vi "ROI grp-Recover Groups array setup.vi"(8 "error in (no error)":errorcluster) -> (0 "error out":errorcluster)   [LabVIEW 2017]
uses:
  ROI Selection Interface/ROI group info cluster.ctl
  Experiment header interface/Typedefs/Save-Load-Save as-Load last enum.ctl
  Global variables/gl_Functional Imaging-Global variables.vi
panel:
  out "Groups setup":T1[](array[typedef]) {"Group region specifier cluster"."Contours"."Type" items=["No Selection", "Point", "Line", "Rectangle", "Oval", "Polygon", "Freehand Region", "Annulus", "Unused2", "Unused3", "Broken Line", "Freehand Line", "Rotated Rectangle"]}
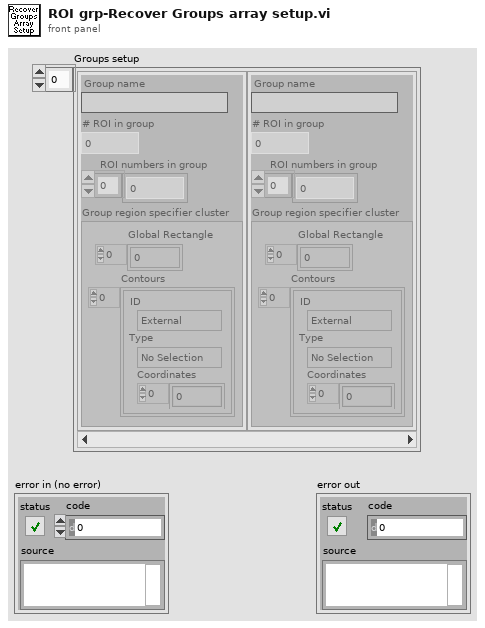
[diagram p1: front panel]
types:
  T1 = typedef "ROI group info cluster.ctl" = cluster{"Group name":string, "# ROI in group":i32, "ROI numbers in group":i32[], "Group region specifier cluster":T2}
  T2 = typedef "ROI Descriptor" = cluster{"Global Rectangle":i32[], "Contours":cluster{"ID":enum32{"External", "Internal"}, "Type":u32, "Coordinates":i32[]}[]}
  T3 = typedef "Save-Load-Save as-Load last enum.ctl" = enum16{"Save file", "Save file as", "Load file", "Load last file"}
  T4 = typedef "Functional Imging UI Refs.ctl" = cluster{"Menu ref":refnum<k9>, "Image control":refnum<vi>, "VI ref":refnum<vi>, "XGrapher":refnum<vi>, "Smoothing":refnum<vi>, "POI Averaging":refnum<vi>, "Normalize":refnum<vi>, "POI data points in each trial":refnum<vi>, "Channel":refnum<vi>, "Experiment data folder path":refnum<vi>, "[ROI vis]":refnum<vi>, "[Groups] visbl":T5, "Group Name":refnum<vi>, "POI index":refnum<vi>, "Trial No.":refnum<vi>, "Intensity Zoom":refnum<vi>, "Trial Cursor Enabled":refnum<vi>, "Number of Trials (ind 1)":refnum<vi>, "Number of Trials (ind 2)":refnum<vi>, "MiniScans Available":refnum<vi>, "POI Available":refnum<vi>, "Defer graph updates":refnum<vi>, "Waveform selector":refnum<vi>, "#of selected POI":refnum<vi>, "#of selected MiniScans":refnum<vi>, "#of selected groups":refnum<vi>, "Max Z-Projection":refnum<vi>, "Z-Plane Selector":refnum<vi>, "Index of miniscan point to visualise":refnum<vi>, "ROI vis. mode":refnum<vi>, "Total # of points":refnum<vi>, "Index of group clicked on":refnum<vi>, "Pane 1":refnum<vi>, "Pane 2":refnum<vi>, "Pane 3":refnum<vi>, "Pane 4":refnum<vi>, "Pane 5":refnum<vi>, "Pane 6":refnum<vi>, "Deselect all ROI":refnum<vi>, "Deselect all groups":refnum<vi>}
  T5 = typedef "Groups array referecne.ctl" = refnum<vi>
  T6 = typedef "Group sel cluster.ctl" = cluster{"Group number":string, "Group Name":string, "Visibility":bool, "Highlight":bool}
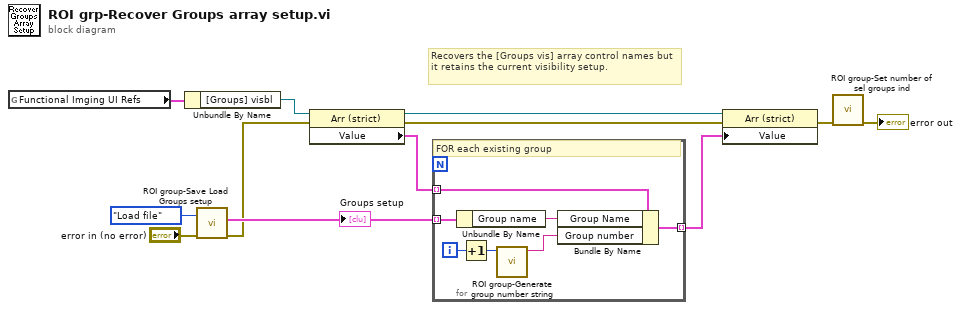
[diagram p0: block diagram]
diagram:
  # "Recovers the [Groups vis] array control names but it retains the current visibility setup."
  n1 = global read "gl_Functional Imaging-Global variables.vi" "Functional Imging UI Refs"() -> (w9:T4)
  n2 = Unbundle By Name(w9) -> ("[Groups] visbl"=w5:T5)
  n3 = call "ROI group-Save Load Groups setup.vi"("error in (no error)"="error in (no error)", "Function"=Save-Load-Save_as-Load_last_enum."Load file") -> ("error out"=w2:errorcluster, "Loaded groups setup"=w7:T1[])  [unwired: 8 in]
  "Groups setup" <- w7
  n4 = property on="Property Node" class="Arr (strict)"(reference=w5, error in=w2) -> (reference out=w4:T5, error out=w3:errorcluster, "Value"=w1:T6[])
  n5 = for {
    tunnel: w7 -> [w19] mode=indexing
    tunnel: [w17] -> w12 mode=indexing
    tunnel: w1 -> [w13] mode=indexing
    i -> [w16]
    # "FOR each existing group"
    n6 = Unbundle By Name(w19) -> ("Group name"=w18:string)
    n7 = Increment(x=w16) -> (x+1=w14:i32)
    n8 = call "ROI group-Generate group number string.vi"("Group number"=w14) -> ("Group number string"=w15:string)  [unwired: 10 in]
    n9 = Bundle By Name(cluster=w13, "Group Name"=w18, "Group number"=w15) -> (w17:T6)
  }
  n10 = property on="Property Node" class="Arr (strict)"(reference=w4, error in=w3, "Value"=w12) -> (error out=w11:errorcluster)  [unwired: 1 out]
  n11 = call "ROI group-Set number of sel groups ind.vi"("error in (no error)"=w11) -> ("error out"=→"error out":errorcluster)  [unwired: 10 in]
